vi "Cursor.vi"(8 "error in (no error)":errorcluster, 9 "disable click? (T)":bool=TRUE, 10 "Top Level VI":string) -> (0 "error out":errorcluster, 3 "Cursor out":refnum<class "Cursor.lvclass">)   [LabVIEW 2023, in "Panel Actor.lvlib" / "Panel.lvlib" / "Cursor.lvclass"]
doc: "Constructs a new Cursor object.\n\n----\nPlease see the following web address for additional documentation and tutorial information:\nhttp://www.mooregoodideas.com/mgi-panel-manager/\n\nAuthor: Derek Trepanier\n\nCopyright (c) 2018, Moore Good Ideas, Inc.\n\nAll rights reserved.\n\nRedistribution and use in source and binary forms, with or without modification, are permitted provided that the following conditions are met:\n\n * Redistributions of source code must retain the above copyright notice, this list of conditions and the following disclaimer.\n * Redistributions in binary form must reproduce the above copyright notice, this list of conditions and the following disclaimer in the documentation and/or other materials provided with the distribution.\n * Neither the name of Moore Good Ideas, Inc. nor the names of its contributors may be used to endorse or promote products derived from this software without specific prior written permission.\n\nTHIS SOFTWARE IS PROVIDED BY THE COPYRIGHT HOLDERS AND CONTRIBUTORS \"AS IS\" AND ANY EXPRESS OR IMPLIED WARRANTIES, INCLUDING, BUT NOT LIMITED TO, THE IMPLIED WARRANTIES OF MERCHANTABILITY AND FITNESS FOR A PARTICULAR PURPOSE ARE DISCLAIMED. IN NO EVENT SHALL THE COPYRIGHT OWNER OR CONTRIBUTORS BE LIABLE FOR ANY DIRECT, INDIRECT, INCIDENTAL, SPECIAL, EXEMPLARY, OR CONSEQUENTIAL DAMAGES (INCLUDING, BUT NOT LIMITED TO, PROCUREMENT OF SUBSTITUTE GOODS OR SERVICES; LOSS OF USE, DATA, OR PROFITS; OR BUSINESS INTERRUPTION) HOWEVER CAUSED AND ON ANY THEORY OF LIABILITY, WHETHER IN CONTRACT, STRICT LIABILITY, OR TORT (INCLUDING NEGLIGENCE OR OTHERWISE) ARISING IN ANY WAY OUT OF THE USE OF THIS SOFTWARE, EVEN IF ADVISED OF THE POSSIBILITY OF SUCH DAMAGE."
uses:
  Cursor.lvclass
  Lookup Actions.ctl
  Cursor.lvclass/Cursor.ctl
  Panel Control Counter/Panel Control Counter.lvclass
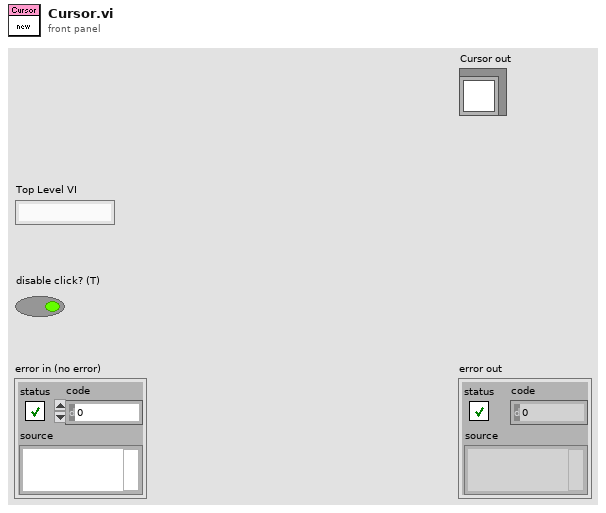
[diagram p1: front panel]
types:
  T1 = typedef "Panel Actor.lvlib/Panel.lvlib/Cursor.lvclass/Lookup Actions.ctl" = enum16{"Init", "Get", "Destroy"}
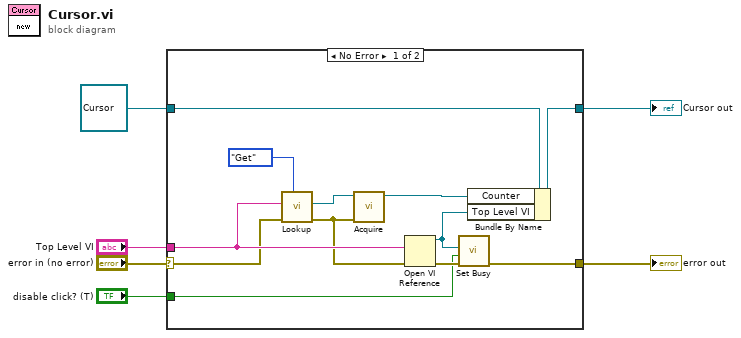
[diagram p0: block diagram]
diagram:
  n1 = case shown="No Error" "error in (no error)" {
    selector: "error in (no error)" -> [w15 w20]
    tunnel: [w13 w20] -> w5
    tunnel: [w12 w19] -> w3
    tunnel: refnum<class "Cursor.lvclass"> refnum ("Cursor in") -> [w18 w19]
    tunnel: "Top Level VI" -> [w16 _]
    tunnel: "disable click? (T)" -> [w7 _]
    frame No Error {
      n2 = call "Lookup.vi"("Action"=Lookup_Actions."Get", "error in (no error)"=w15, "Top Level VI"=w16) -> ("error out"=w8:errorcluster, "Counter"=w11:refnum<class "Panel Control Counter.lvclass">)  [unwired: 7 in]
      n3 = call "Acquire.vi"("error in (no error)"=w8, "Panel Control Counter in"=w11) -> ("Panel Control Counter out"=w10:refnum<class "Panel Control Counter.lvclass">)  [unwired: 8 in, 1 out]
      n4 = Open VI Reference(vi path=w16, error in (no error)=w8) -> (vi reference=w9:refnum<vi>, error out=w14:errorcluster)  [unwired: 4 in]
      n5 = call <vilib>:"Set Busy.vi"("error in (no error)"=w14, "disable click? (T)"=w7, "VI reference (current VI)"=w9) -> ("error out"=w13:errorcluster)  [unwired: 7 in, 1 out]
      n6 = Bundle By Name(cluster=w18, "Counter"=w10, "Top Level VI"=w9) -> (w12:refnum<class "Cursor.lvclass">)
    }
    frame Error {
    }
  }
  "error out" <- w5
  "Cursor out" <- w3
